vi "Read Name.vi"(8 "error in (no error)":errorcluster, 11 "MusicElement in":refnum<class "MusicElement.lvclass">) -> (0 "error out":errorcluster, 2 "Name":string, 3 "MusicElement out":refnum<class "MusicElement.lvclass">)   [LabVIEW 2015, in "MusicElement.lvclass"]
uses:
  MusicElement.lvclass
  MusicElement.lvclass/MusicElement.ctl
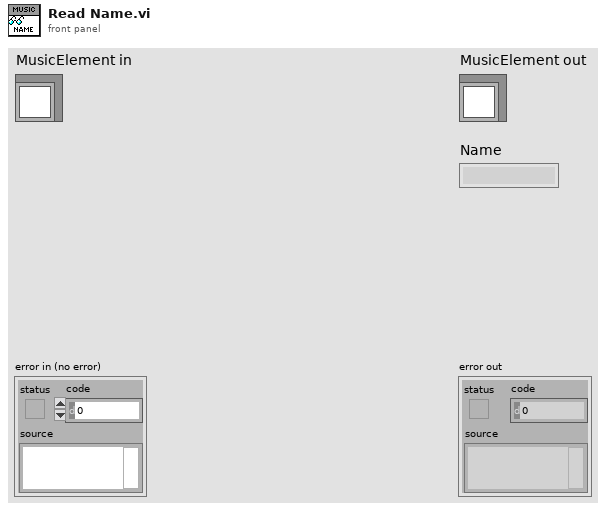
[diagram p1: front panel]
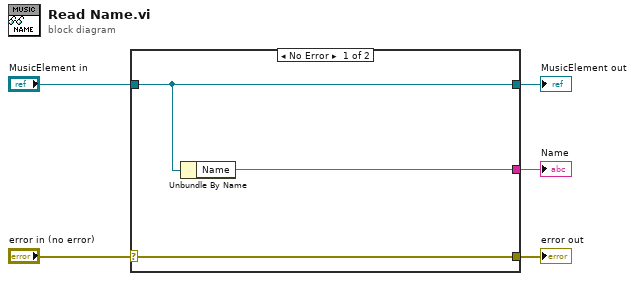
[diagram p0: block diagram]
diagram:
  n1 = case shown="No Error" "error in (no error)" {
    selector: "error in (no error)" -> [w8 w9]
    tunnel: [w8 w9] -> w4
    tunnel: [w7 w10] -> w2
    tunnel: "MusicElement in" -> [w7 w10]
    tunnel: [w6 _] -> w1
    frame No Error {
      n2 = Unbundle By Name(w7) -> ("Name"=w6:string)
    }
    frame Error {
    }
  }
  "error out" <- w4
  "MusicElement out" <- w2
  "Name" <- w1
